vi "Task to String.vi"(11 "Refnum in":refnum<k21>) -> (3 "String":string)   [LabVIEW 2021, in "NI DAQmx_wrapper.lvlib"]
uses:
  NI DAQmx_wrapper.lvlib
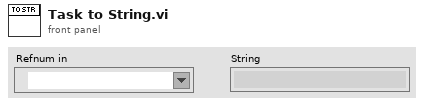
[diagram p1: front panel]
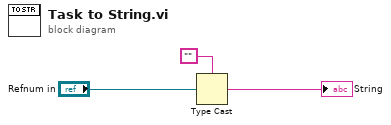
[diagram p0: block diagram]
diagram:
  n1 = Type Cast(type="", x="Refnum in") -> (*(type *) &x=→"String":string)
